vi "uTTA_SwitchPWSTG_PWR.vi"(8 "error in":errorcluster, 9 "Powerstage Power Enable":bool, 11 "VISA Refnum in":refnum<visa-resource-name>) -> (0 "error out":errorcluster, 1 "Powerstage Enabled":bool, 2 "Received":string, 3 "VISA Refnum out":refnum<visa-resource-name>)   [LabVIEW 2021]
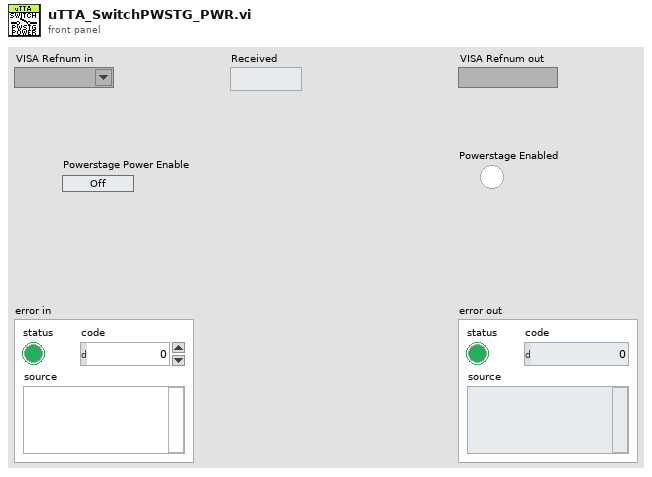
[diagram p1: front panel]
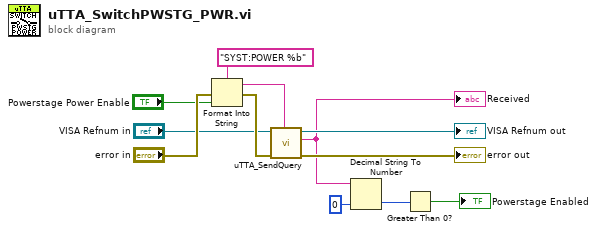
[diagram p0: block diagram]
diagram:
  n1 = Format Into String(format string="SYST:POWER %b", error in="error in", "Powerstage Power Enable") -> (resulting string=w10:string, error out=w12:errorcluster)  [unwired: 1 in]
  n2 = call "uTTA_SendQuery.vi"("Send String"=w10, "error in (no error)"=w12, "VISA Refnum in"="VISA Refnum in") -> ("error out"=→"error out":errorcluster, "Received"=w4:string, "VISA Refnum out"=→"VISA Refnum out":refnum<visa-resource-name>)  [unwired: 6 in]
  "Received" <- w4
  n3 = Decimal String To Number(string=w4, default (0L)=0 ("default (0 I32)")) -> (number=w2:i32)  [unwired: 1 in, 1 out]
  n4 = Greater Than 0?(x=w2) -> (x > 0?=→"Powerstage Enabled":bool)
